vi "remove.vi"(6 "call chain index (1)":i32=1, 7 "vi ref (caller)":refnum<vi>, 8 "error in (no error)":errorcluster) -> (0 "error out":errorcluster)   [LabVIEW 2024, in "summary manager.lvlib"]
uses:
  summary manager.lvlib
  insert or remove.ctl
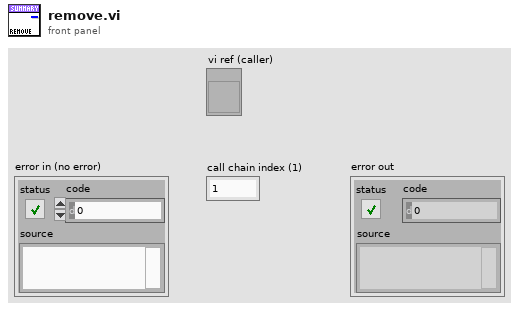
[diagram p1: front panel]
types:
  T1 = typedef "summary manager.lvlib/insert or remove.ctl" = enum16{"insert", "remove"}
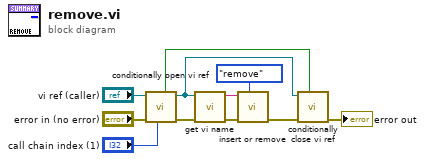
[diagram p0: block diagram]
diagram:
  n1 = call "conditionally open vi ref.vi"("call chain index (1)"="call chain index (1)", "error in (no error)"="error in (no error)", "vi ref in"="vi ref (caller)") -> ("error out"=w8:errorcluster, "vi ref out"=w11:refnum<vi>, "new ref?"=w10:bool)  [unwired: 6 in]
  n2 = call "get vi name.vi"("error in (no error)"=w8, "vi ref"=w11) -> ("error out"=w7:errorcluster, "vi name"=w1:string)  [unwired: 8 in]
  n3 = call "insert or remove.vi"("action"=insert_or_remove."remove", "error in (no error)"=w7, "id"=w1) -> ("error out"=w6:errorcluster)  [unwired: 8 in]
  n4 = call "conditionally close vi ref.vi"("new ref?"=w10, "error in (no error)"=w6, "vi ref"=w11) -> ("error out"=→"error out":errorcluster)  [unwired: 8 in]
